vi "GetResponseData.vi"(11 "string read":string) -> (3 "replaced substring":string)   [LabVIEW 2023]
panel:
  out "x-y":u8
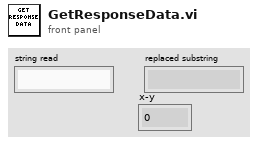
[diagram p1: front panel]
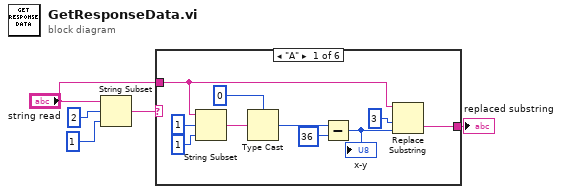
[diagram p0: block diagram]
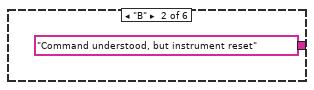
[diagram p2: hidden frame]
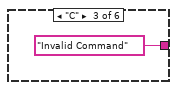
[diagram p3: hidden frame]
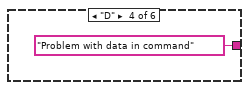
[diagram p4: hidden frame]
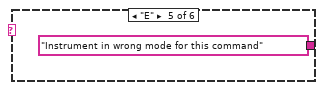
[diagram p5: hidden frame]
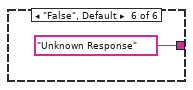
[diagram p6: hidden frame]
diagram:
  n1 = String Subset(string="string read", offset (0)=2, length (rest)=1 ("length (rest)")) -> (substring=w5:string)
  n2 = case shown="\"A\"" w5 {
    tunnel: [w14 "Command understood, but instrument reset" ("replaced substring") "Invalid Command" ("replaced substring") "Problem with data in command" ("replaced substring") "Instrument in wrong mode for this command" ("replaced substring") "Unknown Response" ("replaced substring")] -> w1
    tunnel: "string read" -> [w6 _ _ _ _ _]
    frame "A" {
      n3 = String Subset(string=w6, offset (0)=1, length (rest)=1 ("length (rest)")) -> (substring=w11:string)
      n4 = Type Cast(type=u8 0 ("offset (0)"), x=w11) -> (*(type *) &x=w9:u8)
      n5 = Subtract(x=w9, y=u8 36) -> (x-y=w7:u8)
      "x-y" <- w7
      n6 = Replace Substring(2:w7, 3:3 ("offset (0)"), 5:w6) -> (0:w14:string)  [unwired: 1 in, 1 out]
    }
    frame "B" {
    }
    frame "C" {
    }
    frame "D" {
    }
    frame "E" {
    }
    frame "False", Default {
    }
  }
  "replaced substring" <- w1
